vi "Clusters.vi"() -> ()   [LabVIEW 2018]
panel:
  out "Slide":dbl
  out "Boolean 2":bool
  out "Boolean":bool
  out "Numeric":dbl
  out "Cluster out":T1 {"Slide" scale=0.0..10.0}
  in  "Cluster in":T1 {"Slide" scale=0.0..10.0}
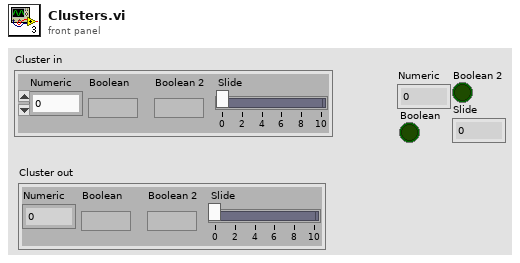
[diagram p1: front panel]
types:
  T1 = cluster{"Numeric":dbl, "Boolean":bool, "Boolean 2":bool, "Slide":dbl}
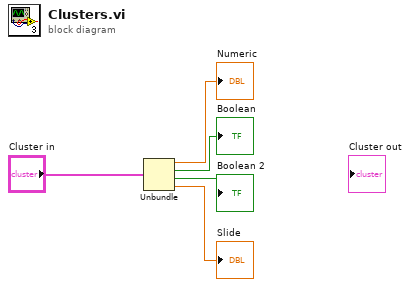
[diagram p0: block diagram]
diagram:
  n1 = Unbundle("Cluster in") -> ("Numeric"=→"Numeric":dbl, "Boolean"=→"Boolean":bool, "Boolean 2"=→"Boolean 2":bool, "Slide"=→"Slide":dbl)
